vi "Read Analogue.vi"(8 "error in (no error)":errorcluster, 11 "KE65XX DMM":refnum<class "Keithley 65XX DMM.lvclass">) -> (0 "error out":errorcluster, 2 "Waveforms":waveform(dbl)[](array[waveform]), 3 "KE65XX DMM out":refnum<class "Keithley 65XX DMM.lvclass">)   [LabVIEW 2025, in "DMM.lvlib" / "Keithley 65XX DMM.lvclass"]
uses:
  Keithley 65XX DMM.lvclass
  Keithley 65XX DMM.lvclass/Keithley 65XX DMM.ctl
  <instrlib>/Keithley 65XX/Drivers/Keithley DMM6500 DAQ6500 Series.lvlib
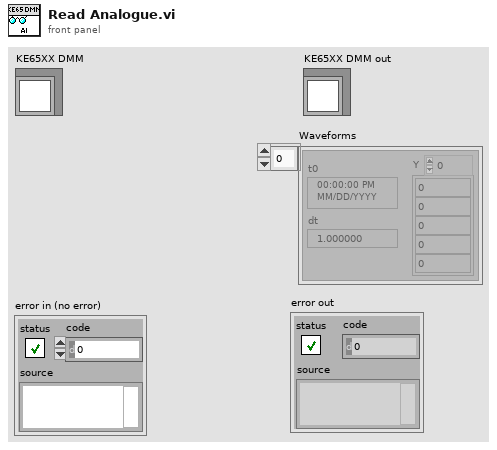
[diagram p1: front panel]
types:
  T1 = typedef "Abstract Engine.lvlibp/Abstract Instrument.lvclass/Channel.ctl" = cluster{"Alias":string, "DataType":enum16{"Anaolg Input", "Waveform"}, "Unit":enum16{"---", "V", "A", "Ohm", "Hz", "uF", "degC", "deg"}, "Upper limit":dbl, "Lower limit":dbl, "Measurement":variant}
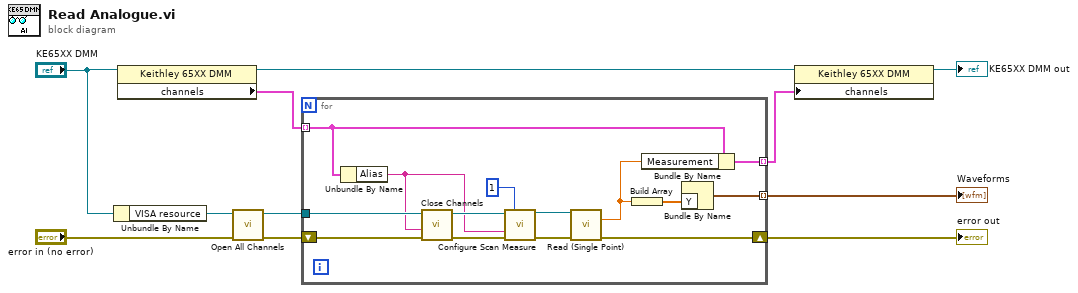
[diagram p0: block diagram]
diagram:
  n1 = Unbundle By Name("KE65XX DMM") -> ("VISA resource"=w10:refnum<visa-resource-name>)
  n2 = property class="Keithley 65XX DMM"(reference="KE65XX DMM") -> (reference out=w5:refnum<class "Keithley 65XX DMM.lvclass">, "channels"=w4:T1[])  [unwired: 1 in, 1 out]
  n3 = call <instrlib>:"Open All Channels.vi"("error in (no error)"="error in (no error)", "VISA resource name"=w10) -> ("error out"=w8:errorcluster, "VISA resource name out"=w9:refnum<visa-resource-name>)  [unwired: 8 in]
  n4 = for {
    tunnel: w9 -> [w25]
    shift-right: [w19] -> w7
    shift-left: w8 -> [w24]
    tunnel: w4 -> [w16] mode=indexing
    tunnel: [w15] -> w2 mode=indexing
    tunnel: [w12] -> w1 mode=indexing
    n5 = Unbundle By Name(w16) -> ("Alias"=w17:string)
    n6 = call <instrlib>:"Close Channels.vi"("error in (no error)"=w24, "Channel List(\"\")"=w17, "VISA resource name"=w25) -> ("error out"=w22:errorcluster, "VISA resource name out"=w23:refnum<visa-resource-name>)  [unwired: 7 in]
    n7 = call <instrlib>:"Configure Scan Measure.vi"("VISA resource name"=w23, "Scan Count (0)"=u32 1, "Channel List(\"\")"=w17, "error in (no error)"=w22) -> ("VISA resource name out"=w21:refnum<visa-resource-name>, "error out"=w20:errorcluster)  [unwired: 10 in]
    n8 = call <instrlib>:"Read (Single Point).vi"("VISA resource name"=w21, "error in (no error)"=w20) -> ("Measurement"=w14:dbl, "error out"=w19:errorcluster)  [unwired: 11 in, 1 out]
    n9 = Build Array(w14) -> (w13:dbl[])
    n10 = Bundle By Name(cluster=w16, "Measurement"=w14) -> (w15:T1)
    n11 = Bundle By Name("Y"=w13) -> (w12:waveform(dbl))  [unwired: 1 in]
  }
  "error out" <- w7
  "Waveforms" <- w1
  n12 = property class="Keithley 65XX DMM"(reference=w5, "channels"=w2) -> (reference out=→"KE65XX DMM out":refnum<class "Keithley 65XX DMM.lvclass">)  [unwired: 1 in, 1 out]
